vi "Put.vi"(8 "error in":errorcluster, 9 "Anything":variant, 10 "endPoint":string, 11 "firebase in":refnum<class "firebase.lvclass">) -> (0 "error out":errorcluster, 2 "Item Name":string, 3 "firebase out":refnum<class "firebase.lvclass">)   [LabVIEW 2019, in "firebase.lvclass"]
uses:
  firebase.lvclass
  8df7efb1-880b-4afd-9d83-a65ebbba9a00.vi
  <vilib>/NI/Advanced HTTP Client/Session.lvclass
  <vilib>/NI/Advanced HTTP Client/Header--Combo Box.ctl
  d9e4e2d6-dd7c-4b59-b05d-e984aa4a9630.vi
  Error Message--cluster.ctl
  8b64f89a-9e96-43c3-a012-814e780b19c4.vi
  <vilib>/JDP Science/JSONtext/JSONtext.lvlib
  Item--cluster.ctl
  <vilib>/NI/Advanced HTTP Client/PUT (Buffer).vi
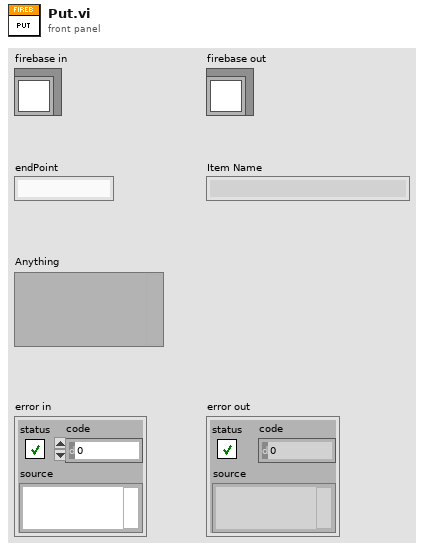
[diagram p1: front panel]
types:
  T1 = typedef "lib_NI_Advanced HTTP Client.lvlib/Session.lvclass/Header--Combo Box.ctl" = string
  T2 = typedef "firebase.lvclass/Success Sign In--cluster.ctl" = cluster{"kind":string, "idToken":string, "email":string, "refreshToken":string, "expiresIn":string, "localId":string, "displayName":string, "registered":bool}
  T3 = typedef "firebase.lvclass/Error Message--cluster.ctl" = cluster{"error":cluster{"code":i32, "message":string, "errors":cluster{"message":string, "domain":string, "reason":string}[]}}
  T4 = typedef "firebase.lvclass/Item--cluster.ctl" = cluster{"name":string}
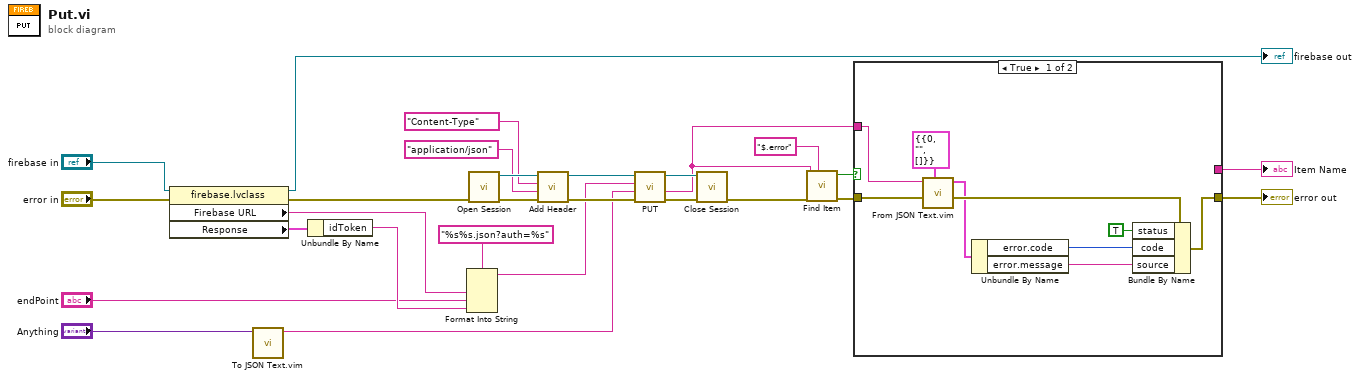
[diagram p0: block diagram]
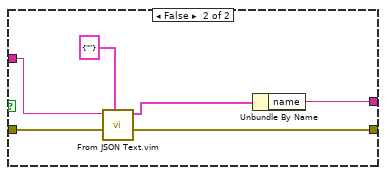
[diagram p2: hidden frame]
diagram:
  n1 = property class="firebase.lvclass"(reference="firebase in", error in="error in") -> (reference out=→"firebase out":refnum<class "firebase.lvclass">, error out=w22:errorcluster, "Firebase URL"=w17:string, "Response"=w4:T2)
  n2 = call "To JSON Text.vim"("Anything"="Anything") -> ("<JSON>"=w10:string)  [unwired: 9 in, 1 out]
  n3 = Unbundle By Name(w4) -> ("idToken"=w3:string)
  n4 = Format Into String(format string="%s%s.json?auth=%s", w17, "endPoint", w3) -> (resulting string=w9:string)  [unwired: 2 in, 1 out]
  n5 = call <vilib>:"Open Session.vi"("error in"=w22) -> ("error out"=w25:errorcluster, "session"=w14:refnum<class "Session.lvclass">)  [unwired: 9 in]
  n6 = call <vilib>:"Add Header.vi"("error in"=w25, "value"="application/json", "header"=T1 "Content-Type", "session in"=w14) -> ("error out"=w24:errorcluster, "session out"=w13:refnum<class "Session.lvclass">)  [unwired: 6 in]
  n7 = call-poly <vilib>:"PUT.vi"("error in"=w24, "buffer"=w10, "url"=w9, "session in"=w13) -> ("error out"=w26:errorcluster, "body"=w6:string, "session out"=w15:refnum<class "Session.lvclass">)  [unwired: 3 in, 2 out]
  n8 = call <vilib>:"Close Session.vi"("error in"=w26, "session"=w15) -> ("error out"=w21:errorcluster)  [unwired: 9 in]
  n9 = call <vilib>:"Find Item.vi"("$Path or Item Name"="$.error", "error in (no error)"=w21, "JSON"=w6) -> ("error out"=w23:errorcluster, "Found"=w7:bool)  [unwired: 5 in, 2 out]
  n10 = case shown="True" w7 {
    tunnel: [w34 w41] -> w20
    tunnel: w23 -> [w36 w42]
    tunnel: w6 -> [w32 w40]
    tunnel: [_ w37] -> w1
    frame True {
      n11 = call "From JSON Text.vim"("Data Type and Default Value"=T3 {"error"={"code"=0, "message"="", "errors"=[]}} ("Error Message"), "error in (no error)"=w36, "JSON"=w32) -> ("error out"=w35:errorcluster, "Data out"=w31:T3)  [unwired: 7 in]
      n12 = Unbundle By Name(w31) -> ("error.code"=w30:i32, "error.message"=w29:string)
      n13 = Bundle By Name(cluster=w35, "status"=TRUE, "code"=w30, "source"=w29) -> (w34:errorcluster)
    }
    frame False {
      n14 = call "From JSON Text.vim"("Data Type and Default Value"=T4 {"name"=""} ("Item"), "error in (no error)"=w42, "JSON"=w40) -> ("error out"=w41:errorcluster, "Data out"=w38:T4)  [unwired: 7 in]
      n15 = Unbundle By Name(w38) -> ("name"=w37:string)
    }
  }
  "error out" <- w20
  "Item Name" <- w1
